vi "PH_USB600x_AnalogReader.panel.vi"(0 "object ref":refnum<vi>, 5 "error in (no error)":errorcluster) -> (19 "error out":errorcluster)   [LabVIEW 2014, in "PH_USB600x_AnalogReader.lvlib"]
doc: "By this VI a ross relais can be monitored and switched. \n\nThe indicators \"CLOSED\", \"OPEN\" and \"SWITCH STATE\" show the value of the Beckhoff-Tag: blue indicates bad tag status reference problems, darkgreen false and lightgreen on. If everything is working fine, \"CLOSED\" and \"SWITCH STATE\" should show the same value, while \"OPEN\" has the opposite value. \n\nThe oval button switches the ross relais. It should be in the same state as the \"SWITCH STATE\" indicator. \n\n\"EXIT\" closes the front panel (GUI), while \"Delete Instance\" disconnects and removes the instance from the PCS.\n\nThis VI has no machine safety relevant logig: there is neither a check of internal conclict nor with other objects, for example conflict with other ross relais. Therefore it must be handled with care and should be operated by well educated operators only. It is forseen exclusively for direct operating and testing of the system. \n\nLicense Agreement for this software:\n\nCopyright (C)\nGesellschaft für Schwerionenforschung, GSI\nPlanckstr. 1\n64291 Darmstadt\nGermany\n\nContact: D.Beck@gsi.de \n\nThis program is free software; you can redistribute it and/or modify it under the terms of the GNU General Public License as published by the Free Software Foundation; either version 2 of the license, or (at your option) any later version.\n\nThis program is distributed in the hope that it will be useful, but WITHOUT ANYW ARRANTY; without even the implied warranty of MERCHANTABILITY or FITNESS FOR A PARTICULAR PURPOSE. See the GNU General License for more details (http://www.gnu.org).\n\nGesellschaft für Schwerionenforschung, GSI\nPlanckstr. 1, 64291 Darmstadt, Germany\nFor all questions and ideas contact: M.Richter@gsi.de, H.Brand@gsi.de or D.Beck@gsi.de.\nLast update: 18-DEC-2002"
uses:
  PH_USB600x_AnalogReader.lvlib
  PH_Basics/PH_StatusHandler/PH_StatusHandler.GUI element.ctl
  PH_USB600x_AnalogReader.Timing.ctl
  CS_Core/CSObj/CSObj.lvlib
  PH_Basics/PH_Common/PH_Common.lvlib
  CS_Core/CSSystem/CSSystemLib/CSSystemLib.lvlib
  PH_Basics/PH_StatusHandler/PH_StatusHandler.lvlib
panel:
  out "Formula":string
  in  "Prdc Interval [s]":dbl
  out "Graph":cluster{"time stamp":timestamp, dbl}[](graph)
  in  "Timing":T1={"Samples per Channel"=1000, "Rate"=1000.0} {"Rate" format="%0.2f"; "Samples per Channel" min=1}
  in  "Timeout [ms]":dbl=1000.0
  in  "Acquire Waveform":bool caption="Acquire\nWaveform"
  out "Status":T2 caption="Enabling State"
  in  "Delete":bool
  in  "Exit":bool
  out "loop counter":i32
  # "PCS"
  # "3.40"
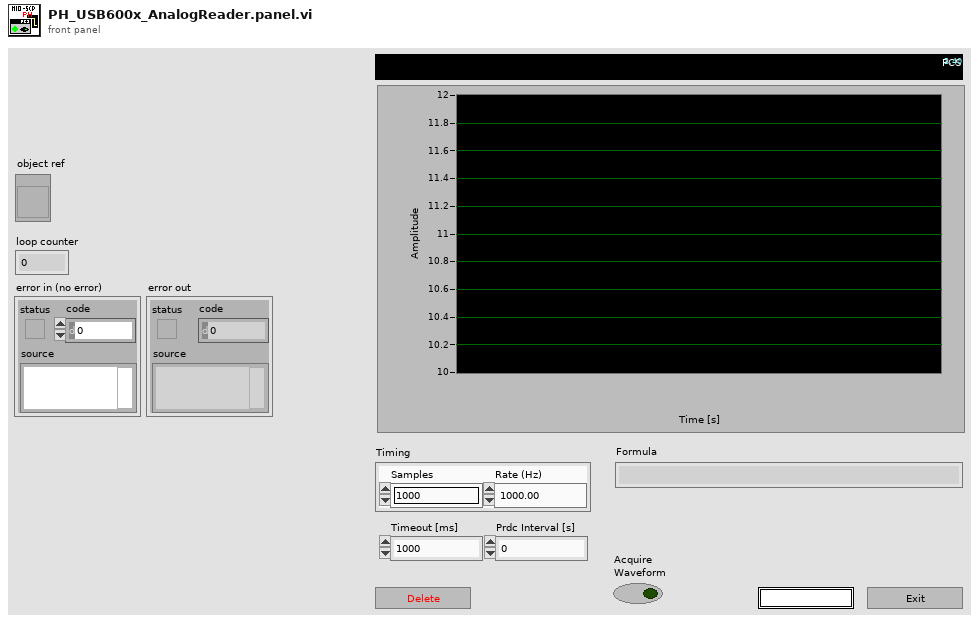
[diagram p1: front panel]
types:
  T1 = typedef "PH_USB600x_AnalogReader.lvlib/PH_USB600x_AnalogReader.Timing.ctl" = cluster{"Samples per Channel":i32, "Rate":dbl}
  T2 = typedef "PH_StatusHandler.lvlib/PH_StatusHandler.GUI element.ctl" = u16
  T3 = typedef "PH_USB600x_AnalogReader.lvlib/PH_USB600x_AnalogReader.i attribute.ctl" = cluster{"GUI Refs":cluster{"Delete":refnum<vi>, "Status":refnum<vi>, "Timeout":refnum<vi>, "Acquire Waveform":refnum<vi>, "Timing":refnum<vi>, "Graph":refnum<vi>, "Prdc Interval":refnum<vi>, "Formula":refnum<vi>}, "Device Settings":cluster{"AIChannel":refnum<k21>, "channelName":string, "Status":T4}, "Timing":T1, "Prdc Interval":dbl, "Lin Scaling":T5, "Data":cluster{"t0":timestamp, dbl}[]}
  T4 = typedef "PH_StatusHandler.lvlib/PH_StatusHandler.Status.ctl" = i16
  T5 = typedef "PH_USB600x_AnalogReader.lvlib/PH_USB600x_AnalogReader.Lin Scaling.ctl" = cluster{"Slope [Unit/V]":dbl, "Offset [Unit]":dbl, "Y-Unit":string, "Y-Label":string}
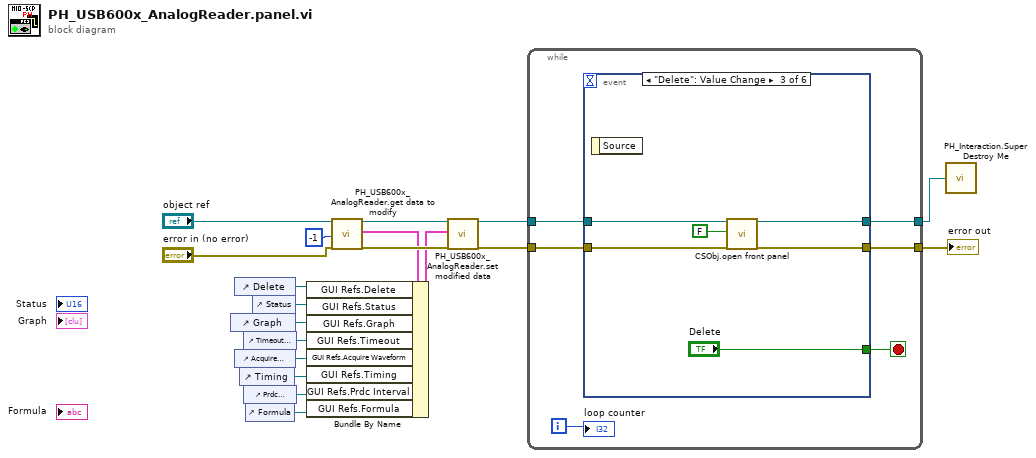
[diagram p0: block diagram]
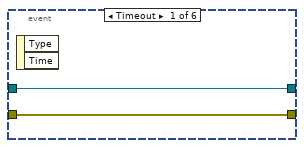
[diagram p2: hidden frame]
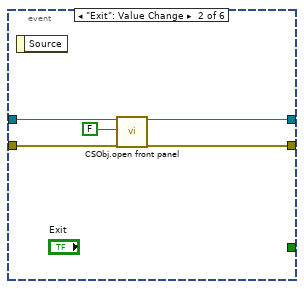
[diagram p3: hidden frame]
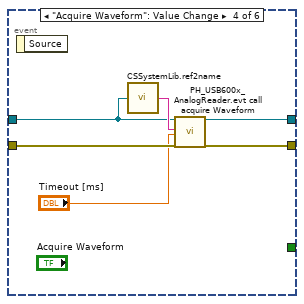
[diagram p4: hidden frame]
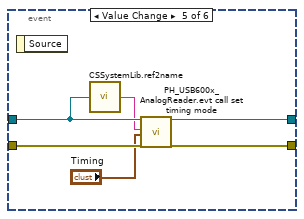
[diagram p5: hidden frame]
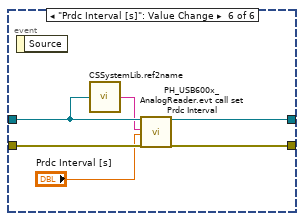
[diagram p6: hidden frame]
diagram:
  n1 = control-ref of="Graph"() -> (w4:refnum<vi>)
  n2 = control-ref of="Delete"() -> (w10:refnum<vi>)
  n3 = control-ref of="Acquire Waveform"() -> (w6:refnum<vi>)
  n4 = control-ref of="Timing"() -> (w5:refnum<vi>)
  n5 = control-ref of="Timeout [ms]"() -> (w7:refnum<vi>)
  n6 = control-ref of="Prdc Interval [s]"() -> (w3:refnum<vi>)
  n7 = control-ref of="Formula"() -> (w2:refnum<vi>)
  n8 = control-ref of="Status"() -> (w1:refnum<vi>)
  n9 = call "PH_USB600x_AnalogReader.get data to modify.vi"("i ref in"="object ref", "ms timeout (10000)"=-1, "error in (no error)"="error in (no error)") -> ("i ref out"=w19:refnum<vi>, "i attribute"=w16:T3, "error out"=w17:errorcluster)  [unwired: 13 in, 1 out]
  n10 = Bundle By Name(cluster=w16, "GUI Refs.Delete"=w10, "GUI Refs.Status"=w1, "GUI Refs.Graph"=w4, "GUI Refs.Timeout"=w7, "GUI Refs.Acquire Waveform"=w6, "GUI Refs.Timing"=w5, "GUI Refs.Prdc Interval"=w3, "GUI Refs.Formula"=w2) -> (w15:T3)
  n11 = call "PH_USB600x_AnalogReader.set modified data.vi"("i ref in"=w19, "i attribute"=w15, "error in (no error)"=w17) -> ("i ref out"=w18:refnum<vi>, "error out"=w13:errorcluster)  [unwired: 15 in]
  n12 = while {
    tunnel: w18 -> [w21]
    tunnel: [w20] -> w9
    tunnel: w13 -> [w23]
    tunnel: [w22] -> w8
    i -> [w24]
    stop <- w25 stop-if-true
    n13 = event shown="[2] \"Delete\": Value Change" {
      selector: _ -> [_ _ _ _ _ _]
      dyn-events: _ -> [_ _ _ _ _ _]
      timeout: _ -> [_ _ _ _ _ _]
      tunnel: [_ _ "Delete" _ _ _] -> w25
      tunnel: w21 -> [w26 w32 w36 w40 w47 w53]
      tunnel: w23 -> [w27 w30 w35 w43 w49 w55]
      tunnel: [w27 w29 w34 w42 w48 w54] -> w22
      tunnel: [w26 w28 w33 w44 w50 w56] -> w20
      event Timeout {
        n14 = event-data() -> ()  [unwired: 1 in, 2 out]
      }
      event "Exit": Value Change {
        n15 = event-data() -> ()  [unwired: 1 in, 1 out]
        n16 = call "CSObj.open front panel.vi"("i ref in"=w32, "frontPanelOpen"=FALSE ("front panel open"), "error in (no error)"=w30) -> ("i ref out"=w28:refnum<vi>, "error out"=w29:errorcluster)  [unwired: 15 in]
      }
      event "Delete": Value Change {
        n17 = event-data() -> ()  [unwired: 1 in, 1 out]
        n18 = call "CSObj.open front panel.vi"("i ref in"=w36, "frontPanelOpen"=FALSE ("front panel open"), "error in (no error)"=w35) -> ("i ref out"=w33:refnum<vi>, "error out"=w34:errorcluster)  [unwired: 15 in]
      }
      event "Acquire Waveform": Value Change {
        n19 = event-data() -> ()  [unwired: 1 in, 1 out]
        n20 = call "CSSystemLib.ref2name.vi"("obj refnum"=w40) -> ("name"=w41:string)
        n21 = call "PH_USB600x_AnalogReader.evt call acquire Waveform.vi"("i ref in"=w40, "Instance"=w41, "Timeout"="Timeout [ms]", "error in"=w43) -> ("i ref out"=w44:refnum<vi>, "error out"=w42:errorcluster)  [unwired: 14 in]
      }
      event Value Change {
        n22 = event-data() -> ()  [unwired: 1 in, 1 out]
        n23 = call "CSSystemLib.ref2name.vi"("obj refnum"=w47) -> ("name"=w46:string)
        n24 = call "PH_USB600x_AnalogReader.evt call set timing mode.vi"("i ref in"=w47, "Instance"=w46, "Timing"="Timing", "error in"=w49) -> ("i ref out"=w50:refnum<vi>, "error out"=w48:errorcluster)  [unwired: 14 in]
      }
      event "Prdc Interval [s]": Value Change {
        n25 = event-data() -> ()  [unwired: 1 in, 1 out]
        n26 = call "CSSystemLib.ref2name.vi"("obj refnum"=w53) -> ("name"=w52:string)
        n27 = call "PH_USB600x_AnalogReader.evt call set Prdc Interval.vi"("i ref in"=w53, "Instance"=w52, "Prdc Interval [s]"="Prdc Interval [s]", "error in"=w55) -> ("i ref out"=w56:refnum<vi>, "error out"=w54:errorcluster)  [unwired: 14 in]
      }
    }
    "loop counter" <- w24
  }
  "error out" <- w8
  n28 = call "PH_Interaction.Super Destroy Me.vi"("i ref out"=w9) -> ()
